vi "MainOrlando.vi"() -> ()   [LabVIEW 2018]
uses:
  <vilib>/addons/zeromq/zmq_context.lvclass
  Channel Rep/Channel Rep.lvclass
  C:/Users/Denis/Desktop/communication-manager/communication-manager/Communication Channel/Communication Channel Folder/Communication Channel.lvclass
  Channel Req/Channel Req.lvclass
  Channel Sub/Channel Sub.lvclass
  Channel Pub/Channel Pub.lvclass
  Communication Channel/Communication Channel Folder/Communication Channel.lvclass
panel:
  in  "Channel Pub.lvclass":refnum<class "Channel Pub.lvclass">
  in  "Channel Sub.lvclass":refnum<class "Channel Sub.lvclass">
  in  "Channel Req.lvclass":refnum<class "Channel Req.lvclass">
  in  "Channel Rep.lvclass":refnum<class "Channel Rep.lvclass">
  out "context":refnum<class "zmq_context.lvclass">
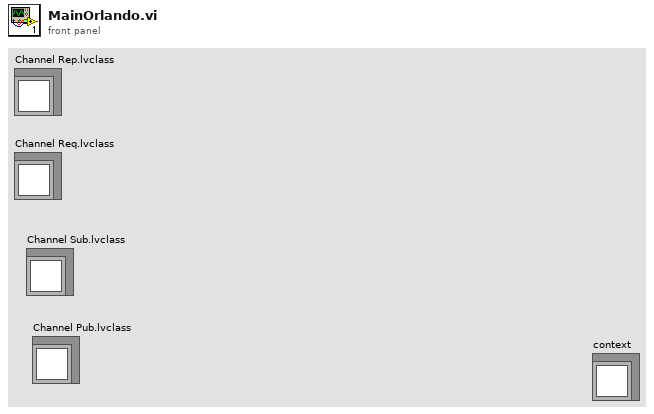
[diagram p1: front panel]
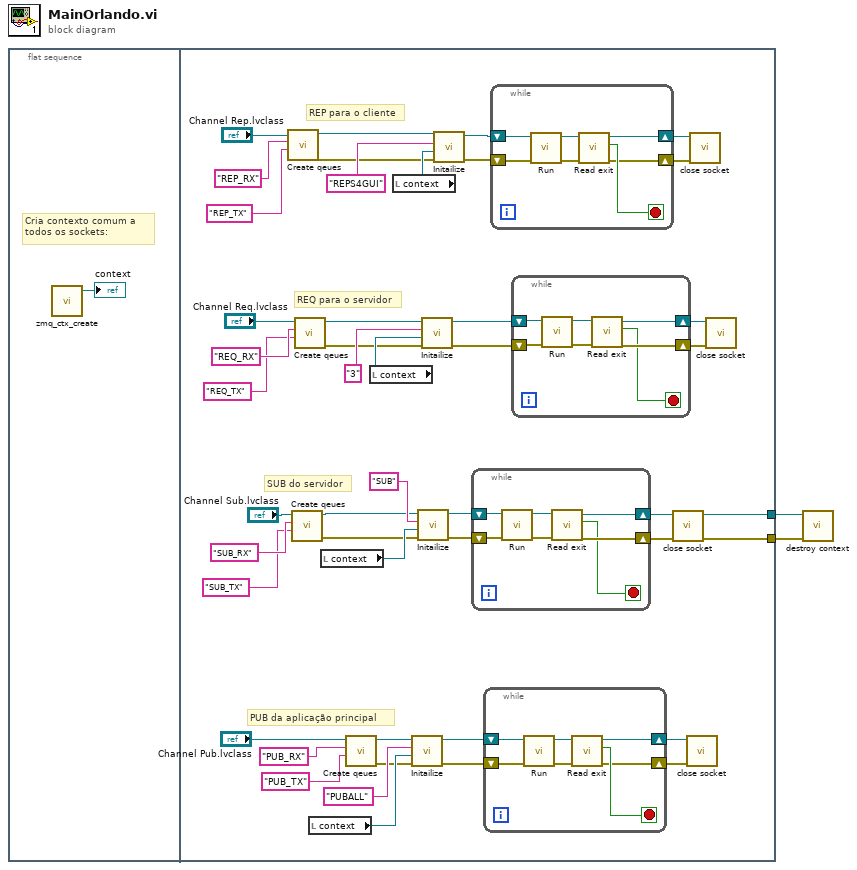
[diagram p0: block diagram]
diagram:
  n1 = flat-sequence {
    tunnel: [w37] -> w2
    tunnel: [w36] -> w1
    frame #0 {
      # "Cria contexto comum a \ntodos os sockets:"
      n2 = call <vilib>:"zmq_ctx_create.vi"() -> ("context out"=→"context":refnum<class "zmq_context.lvclass">)  [unwired: 4 in, 1 out]
    }
    frame #1 {
      # "REP para o cliente"
      # "REQ para o servidor"
      # "PUB da aplicação principal"
      # "SUB do servidor"
      n3 = call "Create qeues.vi"("name qeue Tx"="REP_TX" ("name qeue Rx"), "name qeue Rx"="REP_RX", "Communication Channel in"="Channel Rep.lvclass") -> ("error out"=w12:errorcluster, "Communication Channel out"=w13:refnum<class "Channel Rep.lvclass">)  [unwired: 7 in]
      n4 = call "Create qeues.vi"("name qeue Tx"="SUB_TX" ("name qeue Rx"), "name qeue Rx"="SUB_RX", "Communication Channel in"="Channel Sub.lvclass") -> ("error out"=w33:errorcluster, "Communication Channel out"=w34:refnum<class "Channel Sub.lvclass">)  [unwired: 7 in]
      n5 = call "Create qeues.vi"("name qeue Tx"="REQ_TX" ("name qeue Rx"), "name qeue Rx"="REQ_RX", "Communication Channel in"="Channel Req.lvclass") -> ("error out"=w15:errorcluster, "Communication Channel out"=w16:refnum<class "Channel Req.lvclass">)  [unwired: 7 in]
      n6 = local read "context"() -> (w42:refnum<class "zmq_context.lvclass">)
      n7 = local read "context"() -> (w46:refnum<class "zmq_context.lvclass">)
      n8 = call "Create qeues.vi"("name qeue Tx"="PUB_TX" ("name qeue Rx"), "name qeue Rx"="PUB_RX", "Communication Channel in"="Channel Pub.lvclass") -> ("error out"=w31:errorcluster, "Communication Channel out"=w32:refnum<class "Channel Pub.lvclass">)  [unwired: 7 in]
      n9 = local read "context"() -> (w22:refnum<class "zmq_context.lvclass">)
      n10 = local read "context"() -> (w24:refnum<class "zmq_context.lvclass">)
      n11 = call-dynamic "Initailize.vi"("error in (no error)"=w31, "zeromq.lvlib:ZeroMQ Context"=w42, "Name"="PUBALL", "Channel Pub in"=w32) -> ("error out"=w44:errorcluster, "Channel Pub out"=w45:refnum<class "Channel Pub.lvclass">)  [unwired: 6 in]
      n12 = call-dynamic "Initailize.vi"("error in (no error)"=w33, "zeromq.lvlib:ZeroMQ Context"=w46, "Name"="SUB", "Channel Sub in"=w34) -> ("error out"=w48:errorcluster, "Channel Sub out"=w49:refnum<class "Channel Sub.lvclass">)  [unwired: 6 in]
      n13 = call-dynamic "Initailize.vi"("error in (no error)"=w15, "zeromq.lvlib:ZeroMQ Context"=w22, "Name"="3", "Channel Sub in"=w16) -> ("error out"=w18:errorcluster, "Channel Sub out"=w19:refnum<class "Channel Req.lvclass">)  [unwired: 6 in]
      n14 = call-dynamic "Initailize.vi"("error in (no error)"=w12, "zeromq.lvlib:ZeroMQ Context"=w24, "Name"="REPS4GUI", "Channel Pub in"=w13) -> ("error out"=w20:errorcluster, "Channel Pub out"=w21:refnum<class "Channel Rep.lvclass">)  [unwired: 6 in]
      n15 = while {
        shift-right: [w66] -> w41
        shift-left: w49 -> [w70]
        shift-right: [w65] -> w40
        shift-left: w48 -> [w69]
        stop <- w64 stop-if-true
        n16 = call-dynamic "Run.vi"("error in (no error)"=w69, "Channel Sub in"=w70) -> ("error out"=w67:errorcluster, "Channel Sub out"=w68:refnum<class "Channel Sub.lvclass">)  [unwired: 8 in]
        n17 = call-dynamic "Read exit.vi"("error in (no error)"=w67, "Communication Channel in"=w68) -> ("error out"=w65:errorcluster, "exit"=w64:bool, "Communication Channel out"=w66:refnum<class "Channel Sub.lvclass">)  [unwired: 7 in]
      }
      n18 = while {
        shift-right: [w71] -> w39
        shift-left: w45 -> [w77]
        shift-right: [w72] -> w38
        shift-left: w44 -> [w76]
        stop <- w73 stop-if-true
        n19 = call-dynamic "Run.vi"("error in (no error)"=w76, "Channel Pub in"=w77) -> ("error out"=w74:errorcluster, "Channel Pub out"=w75:refnum<class "Channel Pub.lvclass">)  [unwired: 8 in]
        n20 = call-dynamic "Read exit.vi"("error in (no error)"=w74, "Communication Channel in"=w75) -> ("error out"=w72:errorcluster, "exit"=w73:bool, "Communication Channel out"=w71:refnum<class "Channel Pub.lvclass">)  [unwired: 7 in]
      }
      n21 = while {
        shift-right: [w57] -> w4
        shift-left: w21 -> [w63]
        shift-right: [w58] -> w5
        shift-left: w20 -> [w62]
        stop <- w59 stop-if-true
        n22 = call-dynamic "Run.vi"("error in (no error)"=w62, "Channel Rep in"=w63) -> ("error out"=w60:errorcluster, "Channel Rep out"=w61:refnum<class "Channel Rep.lvclass">)  [unwired: 8 in]
        n23 = call-dynamic "Read exit.vi"("error in (no error)"=w60, "Communication Channel in"=w61) -> ("error out"=w58:errorcluster, "exit"=w59:bool, "Communication Channel out"=w57:refnum<class "Channel Rep.lvclass">)  [unwired: 7 in]
      }
      n24 = while {
        shift-right: [w52] -> w6
        shift-left: w19 -> [w56]
        shift-right: [w51] -> w7
        shift-left: w18 -> [w55]
        stop <- w50 stop-if-true
        n25 = call-dynamic "Run.vi"("error in (no error)"=w55, "Channel Req in"=w56) -> ("error out"=w53:errorcluster, "Channel Req out"=w54:refnum<class "Channel Req.lvclass">)  [unwired: 8 in]
        n26 = call-dynamic "Read exit.vi"("error in (no error)"=w53, "Communication Channel in"=w54) -> ("error out"=w51:errorcluster, "exit"=w50:bool, "Communication Channel out"=w52:refnum<class "Channel Req.lvclass">)  [unwired: 7 in]
      }
      n27 = call "close socket.vi"("error in (no error)"=w40, "Communication Channel in"=w41) -> ("error out"=w36:errorcluster, "Communication Channel out"=w37:refnum<class "Channel Sub.lvclass">)  [unwired: 8 in]
      n28 = call "close socket.vi"("error in (no error)"=w38, "Communication Channel in"=w39) -> ()  [unwired: 8 in, 2 out]
      n29 = call "close socket.vi"("error in (no error)"=w5, "Communication Channel in"=w4) -> ()  [unwired: 8 in, 2 out]
      n30 = call "close socket.vi"("error in (no error)"=w7, "Communication Channel in"=w6) -> ()  [unwired: 8 in, 2 out]
    }
  }
  n31 = call "destroy context.vi"("error in (no error)"=w1, "Communication Channel in"=w2) -> ()  [unwired: 8 in, 2 out]
